vi "Create Engine Session.vi"() -> ()   [LabVIEW 2020]
uses:
  TSnax/Engine/Engine.lvclass
panel:
  in  "Debug?":bool
  out "Same Ref?":bool
  out "VersionString":string
  out "error out":errorcluster
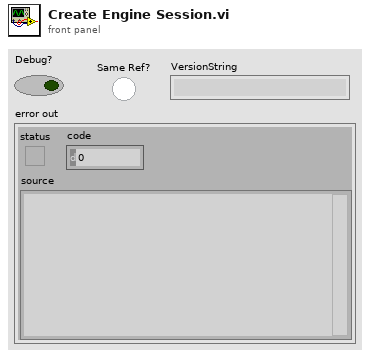
[diagram p1: front panel]
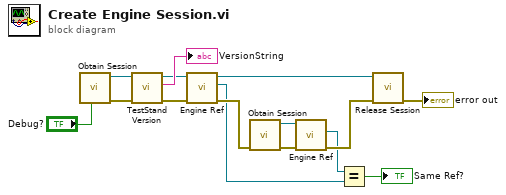
[diagram p0: block diagram]
diagram:
  n1 = call "Obtain Session.vi"("Debug Daemon (Dev Only)"="Debug?") -> ("error out"=w13:errorcluster, "Engine out"=w14:refnum<class "Engine.lvclass">)  [unwired: 9 in]
  n2 = call "TestStand Version.vi"("error in (no error)"=w13, "Engine in"=w14) -> ("error out"=w10:errorcluster, "VersionString"=→"VersionString":string, "Engine out"=w11:refnum<class "Engine.lvclass">)  [unwired: 7 in]
  n3 = call "Engine Ref.vi"("error in (no error)"=w10, "Engine in"=w11) -> ("error out"=w9:errorcluster, "Engine"=w3:refnum<k7>, "Engine out"=w5:refnum<class "Engine.lvclass">)  [unwired: 7 in]
  n4 = call "Obtain Session.vi"("error in (no error)"=w9) -> ("error out"=w8:errorcluster, "Engine out"=w7:refnum<class "Engine.lvclass">)  [unwired: 9 in]
  n5 = call "Engine Ref.vi"("error in (no error)"=w8, "Engine in"=w7) -> ("error out"=w6:errorcluster, "Engine"=w4:refnum<k7>)  [unwired: 7 in, 1 out]
  n6 = Equal?(x=w4, y=w3) -> (x = y?=→"Same Ref?":bool)
  n7 = call "Release Session.vi"("error in (no error)"=w6, "Engine in"=w5) -> ("error out"=→"error out":errorcluster)  [unwired: 9 in]
